vi "DSF.Shared.Configuration.Transfer Group.Check.Transfers.Duplicates.vi"(8 "error in (no error)":errorcluster, 10 "Transfer Configurations in":refnum<class "DSF.Shared.Configuration.Transfer.lvclass">[](array[class]), 11 "Transfer Group Configuration in":refnum<class "DSF.Shared.Configuration.Transfer Group.lvclass">) -> (0 "error out":errorcluster, 2 "Transfer Configurations out":refnum<class "DSF.Shared.Configuration.Transfer.lvclass">[](array[class]), 3 "Transfer Group Configuration out":refnum<class "DSF.Shared.Configuration.Transfer Group.lvclass">)   [LabVIEW 2016, in "DSF.Shared.lvlib" / "DSF.Shared.Configuration.Transfer Group.lvclass"]
uses:
  DSF.Shared.Configuration.Transfer Group.lvclass
  Transfer/DSF.Shared.Configuration.Transfer.lvclass
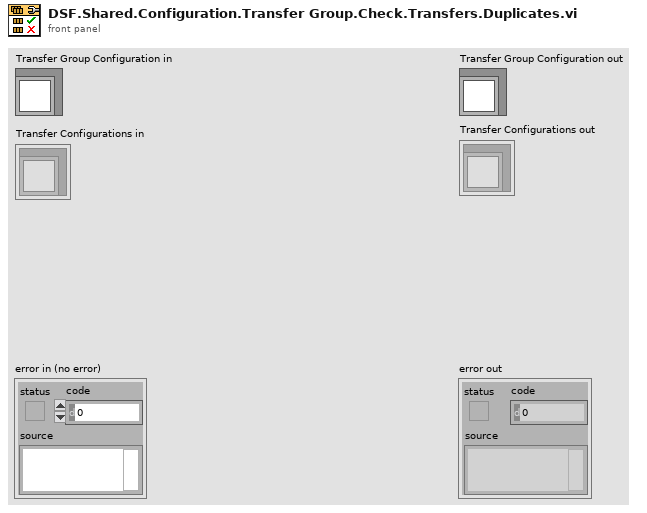
[diagram p1: front panel]
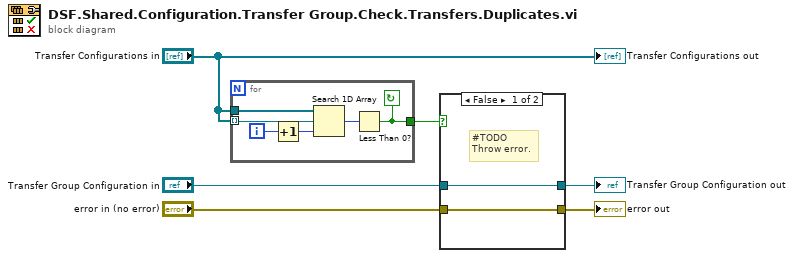
[diagram p0: block diagram]
diagram:
  n1 = for {
    tunnel: [w9] -> w5
    tunnel: "Transfer Configurations in" -> [w8]
    tunnel: "Transfer Configurations in" -> [w7] mode=indexing
    i -> [w12]
    stop <- w9 continue-if-true
    n2 = Increment(x=w12) -> (x+1=w11:i32)
    n3 = Search 1D Array(1D array=w8, element=w7, start index (0)=w11) -> (index of element=w10:i32)
    n4 = Less Than 0?(x=w10) -> (x < 0?=w9:bool)
  }
  n5 = case shown="False" w5 {
    tunnel: "Transfer Group Configuration in" -> [w14 w16]
    tunnel: "error in (no error)" -> [w13 w15]
    tunnel: [w14 w16] -> w2
    tunnel: [w13 w15] -> w1
    frame False {
      # "#TODO\nThrow error."
    }
    frame True {
    }
  }
  "error out" <- w1
  "Transfer Group Configuration out" <- w2
  "Transfer Configurations out" <- "Transfer Configurations in"
